vi "ReadChangedLibrariesLog.vi"(8 "error in (no error)":errorcluster) -> (0 "error out":errorcluster, 2 "ChangedLibraries":string[](array[string]), 3 "ChangedLVFiles":string[](array[string]))   [LabVIEW 2019, in "Hawkeye.lvlib"]
uses:
  Hawkeye.lvlib
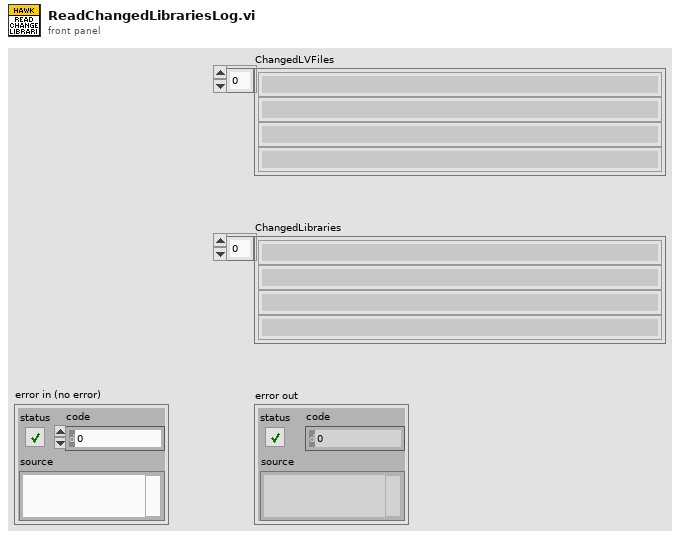
[diagram p1: front panel]
types:
  T1 = enum16{"open", "replace", "create", "open or create", "replace or create", "replace or create with confirmation"}
  T2 = typedef "Hawkeye.lvlib/HawkeyePathConfigs.ctl" = cluster{"GlobalIncludePaths":path[], "GlobalExcludePaths":path[], "BuildSpecsIncludePaths":path[], "ActualDepsIncludePaths":path[], "WorkspacePath":path, "SourceFolderPaths":path[], "ChangedFilesLogpaths":map{string, path}, "CacheRecreateDuration":dbl}
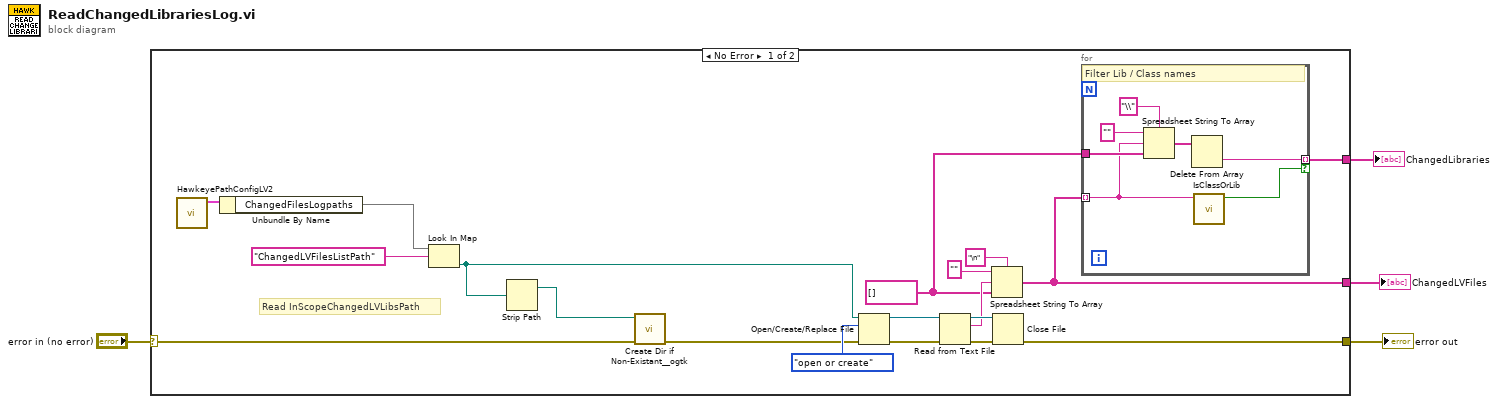
[diagram p0: block diagram]
diagram:
  n1 = case shown="No Error" "error in (no error)" {
    selector: "error in (no error)" -> [w9 w31]
    tunnel: [w7 _] -> w3
    tunnel: [w12 w31] -> w2
    tunnel: [w5 _] -> w1
    frame No Error {
      w6 = string[] []
      # "Read InScopeChangedLVLibsPath"
      n2 = call "HawkeyePathConfigLV2.vi"() -> ("Hawkeye Path Config Out"=w23:T2)  [unwired: 11 in]
      n3 = Unbundle By Name(w23) -> ("ChangedFilesLogpaths"=w21:map{string, path})
      n4 = Look In Map(map=w21, key="ChangedLVFilesListPath") -> (value=w11:path)  [unwired: 1 in, 1 out]
      n5 = Strip Path(path=w11) -> (stripped path=w10:path)  [unwired: 1 out]
      n6 = call <userlib>:"Create Dir if Non-Existant__ogtk.vi"("error in (no error)"=w9, "Directory Path"=w10) -> ("error out"=w8:errorcluster)  [unwired: 7 in, 2 out]
      n7 = Open/Create/Replace File(file path (use dialog)=w11, error in=w8, operation (0:open)=T1."open or create") -> (refnum out=w19:refnum<file>, error out=w18:errorcluster)  [unwired: 3 in, 1 out]
      n8 = Read from Text File(file (use dialog)=w19, error in=w18) -> (refnum out=w17:refnum<file>, text=w15:string, error out=w16:errorcluster)  [unwired: 2 in, 1 out]
      n9 = Spreadsheet String To Array(delimiter (Tab)="\n", format string="", spreadsheet string=w15, array type (2D Dbl)=w6) -> (array=w7:string[])
      n10 = Close File(refnum=w17, error in=w16) -> (error out=w12:errorcluster)  [unwired: 1 out]
      n11 = for {
        tunnel: w7 -> [w24] mode=indexing
        tunnel: w6 -> [w28]
        tunnel: [w26] -> w5 mode=indexing if=w25
        # "Filter Lib / Class names"
        n12 = Spreadsheet String To Array(delimiter (Tab)="\\", format string="", spreadsheet string=w24, array type (2D Dbl)=w28) -> (array=w27:string[])
        n13 = Delete From Array(array=w27) -> (deleted portion=w26:string)  [unwired: 2 in, 1 out]
        n14 = call "IsClassOrLib.vi"("LVFile Name"=w24) -> ("Is LVClass or Library?"=w25:bool)  [unwired: 9 in, 1 out]
      }
    }
    frame Error {
    }
  }
  "ChangedLVFiles" <- w3
  "error out" <- w2
  "ChangedLibraries" <- w1
